vi "SortByElement.vi"(3 "error in (no error)":errorcluster, 4 "String":string, 5 "clEvtReportArrayIn":T1 {"Synx" format="%#_4g"}) -> (0 "error out":errorcluster, 2 "clEvtReportArrayOut":T1 {"Synx" format="%#_4g"})   [LabVIEW 2017, in "AppPlugins.lvlib" / "LSEPlugin.lvclass"]
uses:
  LSEPlugin.lvclass
  EventPlugins/EventPluginBaseClass/TypeDefs/clEvtReportArray.ctl
  EventPlugins/EventPluginBaseClass/TypeDefs/clEvtReport.ctl
  EventPlugins/EventPluginBaseClass/EventPluginBaseClass.lvclass
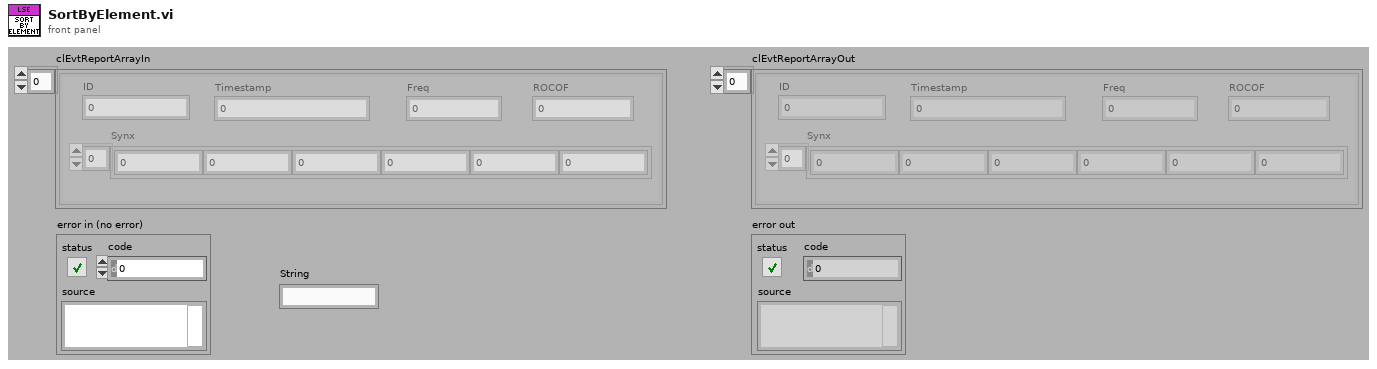
[diagram p1: front panel]
types:
  T1 = typedef "EventPlugins.lvlib/EventPluginBaseClass.lvclass/clEvtReportArray.ctl" = T2[]
  T2 = typedef "EventPlugins.lvlib/EventPluginBaseClass.lvclass/clEvtReport.ctl" = cluster{"Timestamp":dbl, "Synx":cdb[], "Freq":dbl, "ROCOF":dbl, "ID":i16}
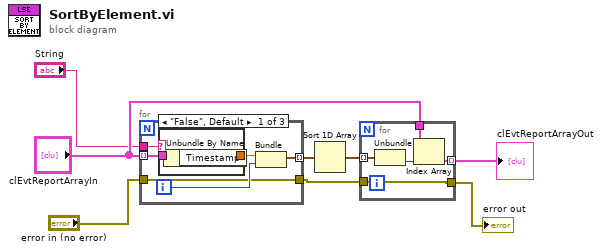
[diagram p0: block diagram]
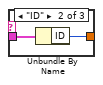
[diagram p2: hidden frame]
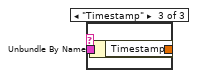
[diagram p3: hidden frame]
diagram:
  n1 = for {
    tunnel: "clEvtReportArrayIn" -> [w14] mode=indexing
    tunnel: [w11] -> w8 mode=indexing
    tunnel: "error in (no error)" -> [w10]
    tunnel: [w10] -> w5
    tunnel: "String" -> [w9]
    i -> [w12]
    n2 = case shown="\"False\", Default" w9 {
      tunnel: w14 -> [w16 w18 w20]
      tunnel: [w15 w17 w19] -> w13
      frame "False", Default {
        n3 = Unbundle By Name(w16) -> ("Timestamp"=w15:dbl)
      }
      frame "ID" {
        n4 = Unbundle By Name(w18) -> ("ID"=w17:i16)
      }
      frame "Timestamp" {
        n5 = Unbundle By Name(w20) -> ("Timestamp"=w19:dbl)
      }
    }
    n6 = Bundle("Timestamp"=w13, w12) -> (w11:cluster{"Timestamp":dbl, i32})  [unwired: 1 in]
  }
  n7 = Sort 1D Array(array=w8) -> (sorted array=w7:cluster{"Timestamp":dbl, i32}[])
  n8 = for {
    tunnel: w7 -> [w25] mode=indexing
    tunnel: "clEvtReportArrayIn" -> [w23]
    tunnel: [w22] -> w3 mode=indexing
    tunnel: w5 -> [w21]
    tunnel: [w21] -> w4
    n9 = Unbundle(w25) -> (w24:i32)  [unwired: 1 out]
    n10 = Index Array(array=w23, index=w24) -> (element=w22:T2)
  }
  "error out" <- w4
  "clEvtReportArrayOut" <- w3
